vi "HandlingEventsInLabVIEW.vi"() -> ()   [LabVIEW 2009]
panel:
  in  "stop":bool
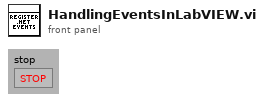
[diagram p1: front panel]
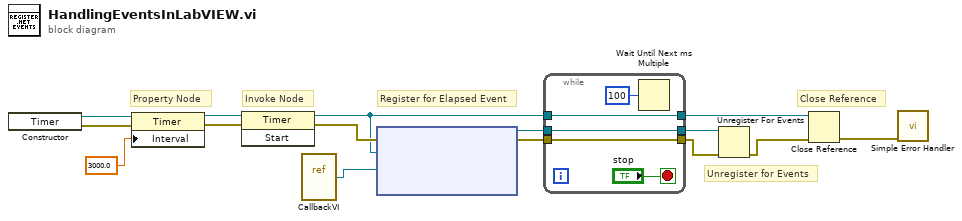
[diagram p0: block diagram]
diagram:
  # "Register for Elapsed Event"
  # "Unregister for Events"
  # "Property Node"
  # "Invoke Node"
  # "Close Reference"
  n1 = constructor class="Timer"() -> (reference out=w15:refnum<k24>, error out=w13:errorcluster)  [unwired: 3 in, 1 out]
  n2 = property class="Timer"(reference=w15, error in=w13, "Interval"=3000.0) -> (reference out=w12:refnum<k24>, error out=w11:errorcluster)
  n3 = invoke class="Timer" method="Start"(reference=w12, error in=w11) -> (reference out=w2:refnum<k24>, error out=w8:errorcluster)  [unwired: 1 in, 1 out]
  n4 = vi-ref "CallbackVI.vi"() -> ("vi reference"=w1:refnum<vi>)
  n5 = node(w8, w2, w1) -> (w6:refnum<k27>, w7:errorcluster)  [unwired: 2 in]
  n6 = while {
    tunnel: [w19] -> w10
    tunnel: w2 -> [w19]
    tunnel: w7 -> [w18]
    tunnel: [w18] -> w4
    tunnel: w6 -> [w17]
    tunnel: [w17] -> w5
    stop <- "stop" stop-if-true
    n7 = Wait Until Next ms Multiple(millisecond multiple=u32 100) -> ()  [unwired: 1 out]
  }
  n8 = Unregister For Events(event registration refnum=w5, error in=w4) -> (error out=w3:errorcluster)
  n9 = Close Reference(reference=w10, error in (no error)=w3) -> (error out=w9:errorcluster)
  n10 = call <vilib>:"Simple Error Handler.vi"("error in (no error)"=w9) -> ()  [unwired: 4 in, 5 out]
